vi "MotionMagicTorqueCurrentFOC Setter.vi"(0 "DeviceReference":T1, 1 "Slot":i32, 2 "LimitForwardMotion":bool, 3 "Update Frequency (Hz)":dbl=100.0, 5 "StopSendingOtherRequests":bool=TRUE, 7 "Position":dbl, 9 "FeedForward":dbl, 12 "OverrideCoastDurNeutral":bool, 13 "LimitReverseMotion":bool) -> (4 "DeviceReference Out":T1)   [LabVIEW 2023]
doc: "Requests Motion Magic® to target a final position using a motion profile. Users can optionally provide a torque current feedforward.\nMotion Magic® produces a motion profile in real-time while attempting to honor the Cruise Velocity, Acceleration, and Jerk value specified via the Motion Magic® configuration values. This control mode does not use the Expo_kV or Expo_kA configs. Target position can be changed on-the-fly and Motion Magic® will do its best to adjust the profile. This control mode is based on torque current, so relevant closed-loop gains will use Amperes for the numerator."
uses:
  Users/Cory/Documents/PhoenixPro-LabVIEW-Generation/controls/DeviceReference.ctl
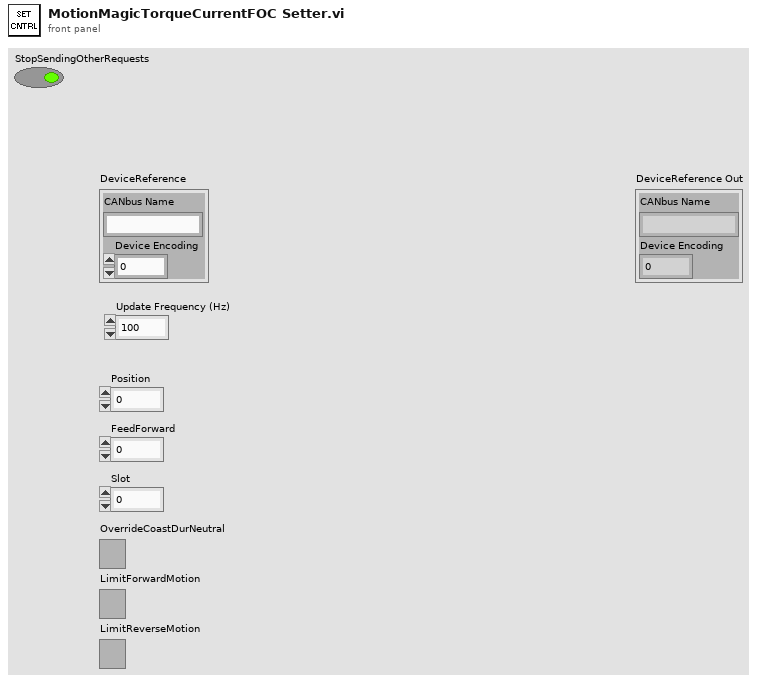
[diagram p1: front panel]
types:
  T1 = typedef "DeviceReference.ctl" = cluster{"CANbus Name":string, "Device Encoding":u32}
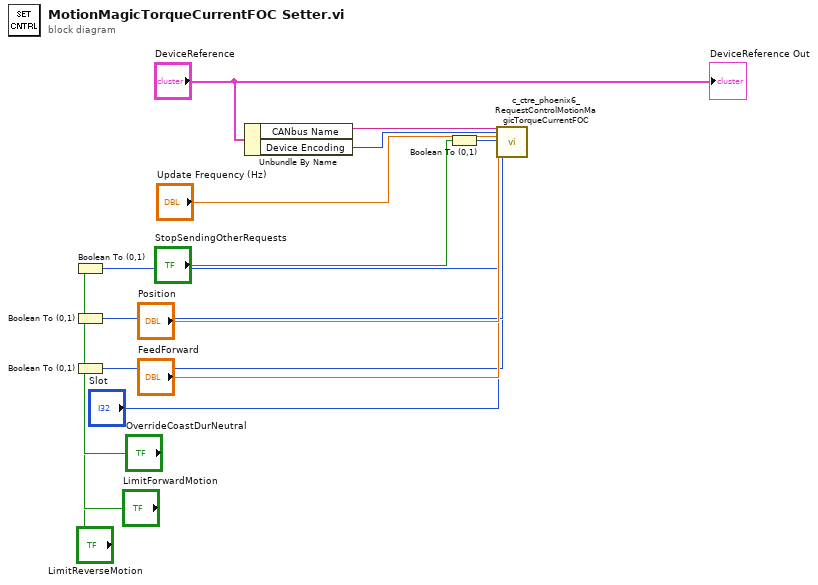
[diagram p0: block diagram]
diagram:
  n1 = Boolean To (0,1)(Boolean="OverrideCoastDurNeutral") -> (0, 1=w5:i16)
  n2 = Boolean To (0,1)(Boolean="LimitForwardMotion") -> (0, 1=w3:i16)
  n3 = Boolean To (0,1)(Boolean="LimitReverseMotion") -> (0, 1=w1:i16)
  n4 = Unbundle By Name("DeviceReference") -> ("CANbus Name"=w14:string, "Device Encoding"=w13:u32)
  n5 = Boolean To (0,1)(Boolean="StopSendingOtherRequests") -> (0, 1=w10:i16)
  n6 = call <vilib>:"c_ctre_phoenix6_RequestControlMotionMagicTorqueCurrentFOC.vi"("String 2"=w14, "Numeric 2"=w13, "Numeric 3"="Update Frequency (Hz)", "Numeric 4"=w10, "Numeric 5"="Position", "Numeric 6"="FeedForward", "Numeric 7"="Slot", "Numeric 8"=w5, "Numeric 9"=w3, "Numeric 10"=w1) -> ()  [unwired: 16 in, 2 out]
  "DeviceReference Out" <- "DeviceReference"
